vi "aptmotorcontrol.vi"() -> ()   [LabVIEW 2013]
panel:
  out "pfPosition 3":sgl
  out "pfPosition 2":sgl
  in  "Serial 3":i32=90848556
  in  "MG17Motor 3":refnum<k7>(container)
  in  "Serial 2":i32=90848555
  in  "MG17Motor 2":refnum<k7>(container)
  out "pfPosition":sgl
  in  "MG17Motor":refnum<k7>(container)
  in  "stop":bool
  in  "Serial":i32=90848557
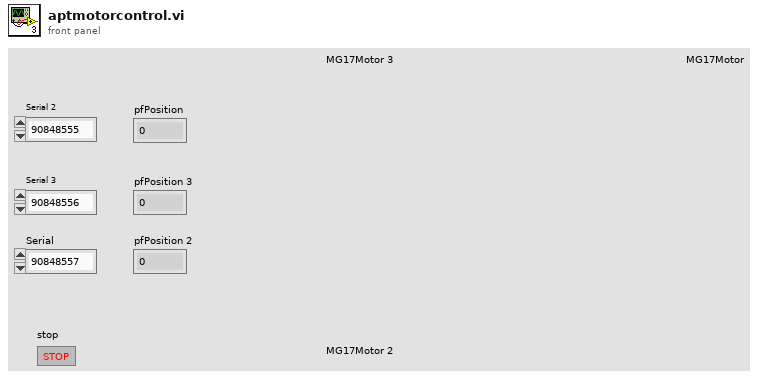
[diagram p1: front panel]
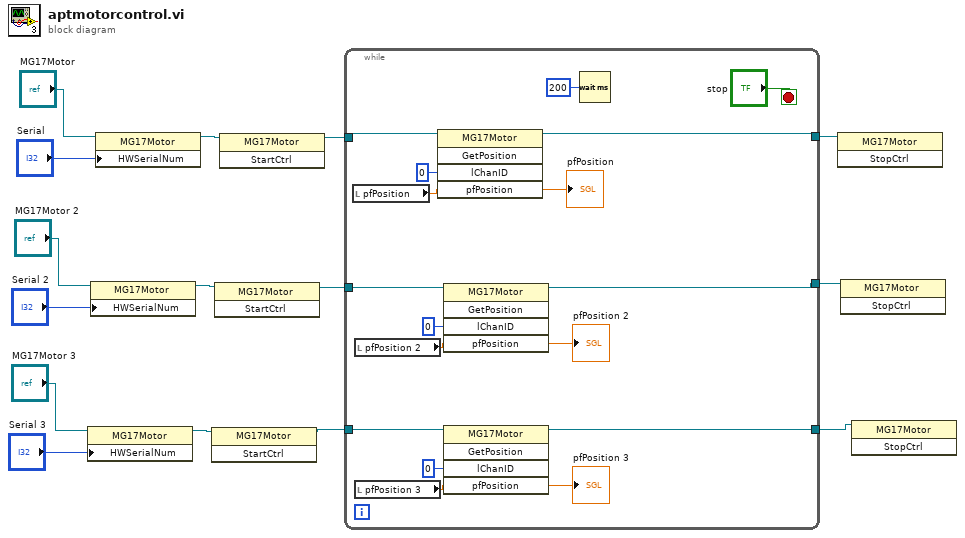
[diagram p0: block diagram]
diagram:
  n1 = property class="MG17Motor"(reference="MG17Motor 3", "HWSerialNum"="Serial 3") -> (reference out=w5:refnum<k7>)  [unwired: 1 in, 1 out]
  n2 = property class="MG17Motor"(reference="MG17Motor 2", "HWSerialNum"="Serial 2") -> (reference out=w8:refnum<k7>)  [unwired: 1 in, 1 out]
  n3 = property class="MG17Motor"(reference="MG17Motor", "HWSerialNum"="Serial") -> (reference out=w11:refnum<k7>)  [unwired: 1 in, 1 out]
  n4 = invoke class="MG17Motor" method="StartCtrl"(reference=w5) -> (reference out=w2:refnum<k7>)  [unwired: 2 in, 2 out]
  n5 = invoke class="MG17Motor" method="StartCtrl"(reference=w8) -> (reference out=w4:refnum<k7>)  [unwired: 2 in, 2 out]
  n6 = invoke class="MG17Motor" method="StartCtrl"(reference=w11) -> (reference out=w13:refnum<k7>)  [unwired: 2 in, 2 out]
  n7 = while {
    tunnel: w13 -> [w31]
    tunnel: [w30] -> w12
    tunnel: w4 -> [w22]
    tunnel: [w21] -> w3
    tunnel: w2 -> [w17]
    tunnel: [w16] -> w1
    stop <- "stop" stop-if-true
    n8 = local read "pfPosition"() -> (w27:sgl)
    n9 = local read "pfPosition 2"() -> (w25:sgl)
    n10 = local read "pfPosition 3"() -> (w18:sgl)
    n11 = invoke class="MG17Motor" method="GetPosition"(reference=w31, "lChanID"=0, "pfPosition"=w27) -> (reference out=w30:refnum<k7>, "pfPosition"=→"pfPosition":sgl)  [unwired: 2 in, 3 out]
    n12 = invoke class="MG17Motor" method="GetPosition"(reference=w22, "lChanID"=0, "pfPosition"=w25) -> (reference out=w21:refnum<k7>, "pfPosition"=→"pfPosition 2":sgl)  [unwired: 2 in, 3 out]
    n13 = invoke class="MG17Motor" method="GetPosition"(reference=w17, "lChanID"=0, "pfPosition"=w18) -> (reference out=w16:refnum<k7>, "pfPosition"=→"pfPosition 3":sgl)  [unwired: 2 in, 3 out]
    n14 = Wait (ms)(milliseconds to wait=u32 200) -> ()  [unwired: 1 out]
  }
  n15 = invoke class="MG17Motor" method="StopCtrl"(reference=w12) -> ()  [unwired: 2 in, 3 out]
  n16 = invoke class="MG17Motor" method="StopCtrl"(reference=w3) -> ()  [unwired: 2 in, 3 out]
  n17 = invoke class="MG17Motor" method="StopCtrl"(reference=w1) -> ()  [unwired: 2 in, 3 out]
